vi "LaunchConfigVIs.vi"(8 "Error In":errorcluster, 10 "Device Name":string, 11 "Module Name":string) -> (0 "Error Out":errorcluster)   [LabVIEW 2011]
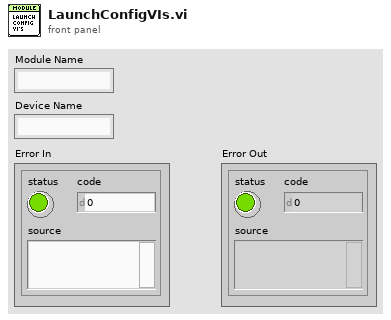
[diagram p1: front panel]
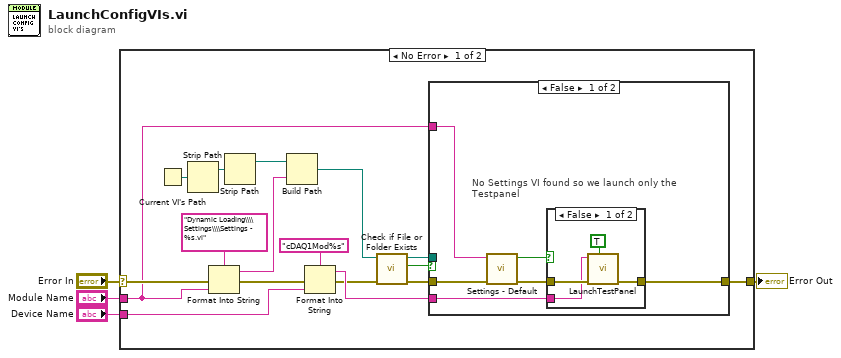
[diagram p0: block diagram]
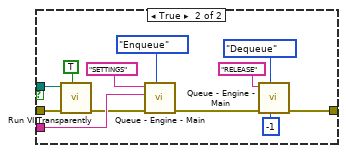
[diagram p3: hidden frame]
diagram:
  n1 = case shown="No Error" "Error In" {
    selector: "Error In" -> [w16 w45]
    tunnel: "Module Name" -> [w5 _]
    tunnel: [w15 w45] -> w3
    tunnel: "Device Name" -> [w13 _]
    frame No Error {
      n2 = Current VI's Path() -> (path=w21:path)
      n3 = Strip Path(path=w21) -> (stripped path=w20:path)  [unwired: 1 out]
      n4 = Format Into String(format string="Dynamic Loading\\\\Settings\\\\Settings - %s.vi", error in=w16, w5) -> (resulting string=w17:string, error out=w7:errorcluster)  [unwired: 1 in]
      n5 = Strip Path(path=w20) -> (stripped path=w19:path)  [unwired: 1 out]
      n6 = Build Path(base path=w19, name or relative path=w17) -> (appended path=w11:path)
      n7 = Format Into String(format string="cDAQ1Mod%s", error in=w7, w13) -> (resulting string=w12:string, error out=w6:errorcluster)  [unwired: 1 in]
      n8 = call <vilib>:"Check if File or Folder Exists.vi"("error in (no error)"=w6, "path"=w11) -> ("error out"=w10:errorcluster, "file or folder exists?"=w8:bool, "dup path"=w9:path)  [unwired: 7 in]
      n9 = case shown="False" w8 {
        tunnel: [w27 w34] -> w15
        tunnel: w12 -> [w24 w42]
        tunnel: w10 -> [w26 w40]
        tunnel: w9 -> [_ w39]
        tunnel: w5 -> [w22 _]
        frame False {
          # "No Settings VI found so we launch only the\nTestpanel"
          n10 = call "Settings - Default.vi"("Error In"=w26, "Module Name In"=w22) -> ("Error Out"=w25:errorcluster, "Cancelled?"=w23:bool)  [unwired: 8 in]
          n11 = case shown="False" w23 {
            tunnel: [w31 w32] -> w27
            tunnel: w25 -> [w29 w32]
            tunnel: w24 -> [w28 _]
            frame False {
              n12 = call "LaunchTestPanel.vi"("Wait Until Completion (T)?"=TRUE, "Error In"=w29, "Device name In"=w28) -> ("Error Out"=w31:errorcluster)  [unwired: 8 in]
            }
            frame True {
            }
          }
        }
        frame True {
          n13 = call "Run VI Transparently.vi"("Run Transparently? (T)"=TRUE, "error in"=w40, "vi path"=w39) -> ("error out"=w41:errorcluster)  [unwired: 8 in]
          n14 = call "Queue - Engine - Main.vi"("Operation"=enum16{"Enqueue", "Dequeue", "Flush", "Release"}."Enqueue", "error in"=w41, "Queue Data In"=w42, "Queue Name In"="SETTINGS") -> ("error out"=w35:errorcluster)  [unwired: 5 in, 2 out]
          n15 = call "Queue - Engine - Main.vi"("timeout in ms (-1)"=-1, "Operation"=enum16{"Enqueue", "Dequeue", "Flush", "Release"}."Dequeue", "error in"=w35, "Queue Name In"="RELEASE" ("Queue Data In")) -> ("error out"=w34:errorcluster)  [unwired: 5 in, 2 out]
        }
      }
    }
    frame Error {
    }
  }
  "Error Out" <- w3
